vi "Reduce Keys to 1D and Unique set.vi"(8 "error in (no error)":errorcluster, 11 "Keys":refnum<class "2D Array u32.lvclass">) -> (0 "error out":errorcluster, 2 "Reduced Keys":refnum<class "1D Array u32.lvclass">, 3 "Unique Keys":refnum<class "1D Array u32.lvclass">)   [LabVIEW 2020, in "G2CPU Line Profile.lvlib"]
uses:
  G2CPU Line Profile.lvlib
  <vilib>/Natan Biesmans/G2CPU GPU and CPU HPC Toolkit/G2CPU Libraries/Arrays/2DArray/u32/2D Array u32.lvclass
  C:/Program Files/National Instruments/LabVIEW 2025/vi.lib/Natan Biesmans/G2CPU GPU and CPU HPC Toolkit/G2CPU Libraries/Arrays/Array/Array Prototype.lvclass
  <vilib>/Natan Biesmans/G2CPU GPU and CPU HPC Toolkit/G2CPU Libraries/Arrays/1DArray/u32/1D Array u32.lvclass
  <vilib>/Natan Biesmans/G2CPU GPU and CPU HPC Toolkit/G2CPU Libraries/Arrays/Array/Array Prototype.lvclass/Array Prototype.ctl
  998b56e5-9620-4ecc-a2fe-a87db3d41caf.vi
  db84f0ca-2980-4c20-933d-5a6197a7408a.vi
  <vilib>/Natan Biesmans/G2CPU GPU and CPU HPC Toolkit/G2CPU Libraries/Arrays/Array/G2CPU Get Array Pointer.vi
  998b56e5-9620-4ecc-a2fe-a87db3d41caf.vi/008596a2-72c7-4b94-8d63-a430db0cac39.vi
  998b56e5-9620-4ecc-a2fe-a87db3d41caf.vi/d781c0aa-35dc-4978-ac14-8fc3832ba4f0.vi
  998b56e5-9620-4ecc-a2fe-a87db3d41caf.vi/5ea8fe8e-4ffc-4d1c-84a0-6eba72fe9718.vi
  998b56e5-9620-4ecc-a2fe-a87db3d41caf.vi/e2c9d363-485e-46f6-8192-2d8aa165dabd.vi
  998b56e5-9620-4ecc-a2fe-a87db3d41caf.vi/677e326b-dc8f-4d68-b1d9-971c0162f72d.vi
  db84f0ca-2980-4c20-933d-5a6197a7408a.vi/c0beb570-c734-45d1-92b7-5f6c2717fc31.vi
  <vilib>/Natan Biesmans/G2CPU GPU and CPU HPC Toolkit/ArrayFire Driver/VIs/imax.vi
  <vilib>/Natan Biesmans/G2CPU GPU and CPU HPC Toolkit/G2CPU Libraries/Arrays/SubVI/RemoveReducedDimensionForReorder.vi
  <vilib>/Natan Biesmans/G2CPU GPU and CPU HPC Toolkit/ArrayFire Driver/VIs/reorder.vi
  <vilib>/Natan Biesmans/G2CPU GPU and CPU HPC Toolkit/ArrayFire Driver/VIs/release array.vi
  <vilib>/Natan Biesmans/G2CPU GPU and CPU HPC Toolkit/G2CPU Libraries/Arrays/Array/G2CPU Set Array Pointer.vi
  <vilib>/Natan Biesmans/G2CPU GPU and CPU HPC Toolkit/ArrayFire Driver/VIs/set unique.vi
  <vilib>/Natan Biesmans/G2CPU GPU and CPU HPC Toolkit/G2CPU Libraries/Arrays/Array/Array Prototype.lvclass
  <vilib>/Natan Biesmans/G2CPU GPU and CPU HPC Toolkit/G2CPU Libraries/Arrays/DataTypes/U32/U32.lvclass
  <vilib>/Natan Biesmans/G2CPU GPU and CPU HPC Toolkit/G2CPU Libraries/Arrays/2DArray/2D Array Prototype.lvclass
  <vilib>/Natan Biesmans/G2CPU GPU and CPU HPC Toolkit/G2CPU Libraries/Arrays/1DArray/1D Array Prototype.lvclass
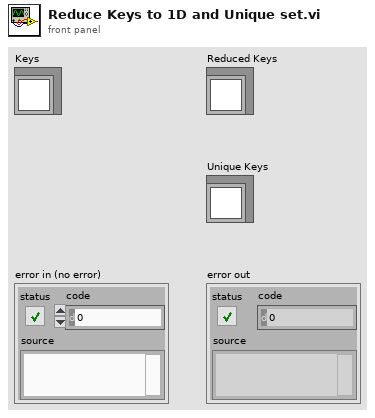
[diagram p1: front panel]
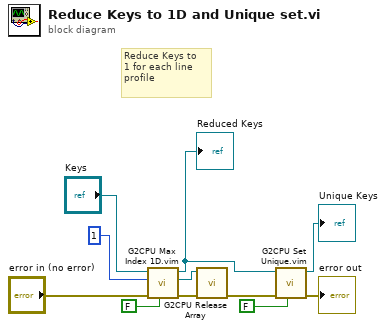
[diagram p0: block diagram]
diagram:
  # "Reduce Keys to\n1 for each line profile"
  n1 = call "G2CPU Max Index 1D.vim"("Auto Release (Enabled)"=FALSE, "error in (no error)"="error in (no error)", "dim"=1, "Array First"="Keys") -> ("error out"=w2:errorcluster, "Array idx"=w1:refnum<class "1D Array u32.lvclass">, "Array out"=w7:refnum<class "1D Array u32.lvclass">)  [unwired: 5 in]
  "Reduced Keys" <- w7
  n2 = call <vilib>:"G2CPU Release Array.vi"("error in (no error)"=w2, "Array in"=w1) -> ("error out"=w4:errorcluster)  [unwired: 9 in]
  n3 = call "G2CPU Set Unique.vim"("Auto Release (Enabled)"=FALSE, "error in (no error)"=w4, "Array in"=w7) -> ("error out"=→"error out":errorcluster, "Array Result"=→"Unique Keys":refnum<class "1D Array u32.lvclass">)  [unwired: 7 in]
